vi "Message assembler for F-70.vi"(11 "command":string="ID1") -> (3 "complete message":string)   [LabVIEW 2021, in "F-70 driver.lvlib"]
doc: "Concatenates a \"$\" as starting character, a command message, its checksum, and ending character \"\\r\".\nInput: just a command message\nOutput: complete message - ready to be send to compressor"
uses:
  F-70 driver.lvlib
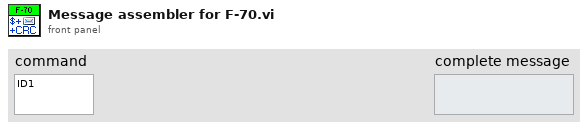
[diagram p1: front panel]
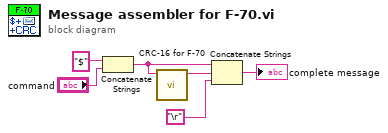
[diagram p0: block diagram]
diagram:
  n1 = Concatenate Strings("$" ("cmd 3"), "command") -> (w4:string)
  n2 = call "CRC-16 for F-70.vi"("DATA PACKET"=w4) -> ("CRC-16 H-str"=w3:string)  [unwired: 4 in, 2 out]
  n3 = Concatenate Strings(w4, w3, "\r") -> (→"complete message":string)
